vi "PQfetchResultDataNotrans.vi"(8 "error in":errorcluster, 10 "res":u64, 11 "conn":u64) -> (0 "error out":errorcluster, 1 "Data":string[][](array[string]), 2 "res_out":u64, 3 "conn_out":u64, 4 "PQnFields":i64, 6 "PQnTuples":i64)   [LabVIEW 2019, in "libpqutility64.lvlib"]
doc: "Fetch Result Data from DatabaseRequest into String Array.\nSee PostgreSQL c-lib doku for further information."
uses:
  libpqutility64.lvlib
  libpqlv64/libpqlv64.lvlib
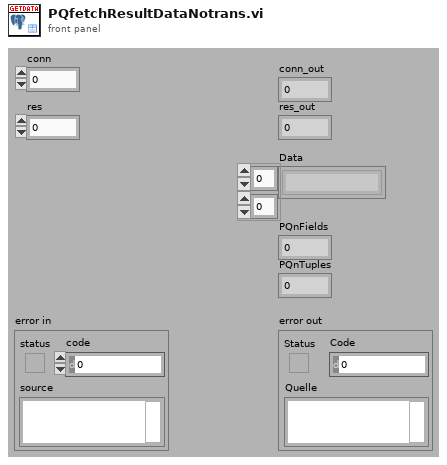
[diagram p1: front panel]
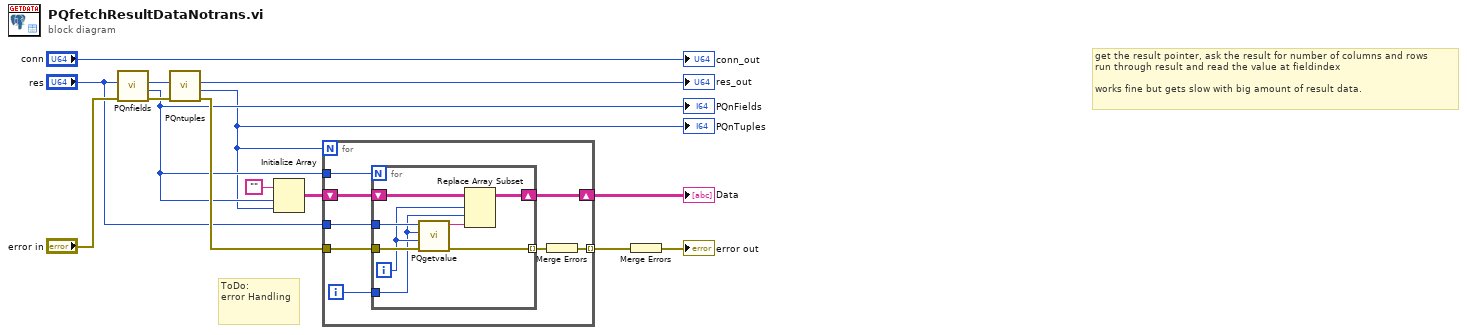
[diagram p0: block diagram]
diagram:
  # "ToDo:\nerror Handling"
  # "get the result pointer, ask the result for number of columns and rows\nrun through result and read the value at fieldindex\n\nworks fine but gets slow with big amount of result data."
  n1 = call "PQnfields.vi"("error in (no error)"="error in", "res"="res") -> ("error out"=w12:errorcluster, "PQnFields"=w6:i64, "res out"=w3:u64)  [unwired: 7 in]
  "PQnFields" <- w6
  n2 = call "PQntuples.vi"("error in (no error)"=w12, "res"=w3) -> ("error out"=w11:errorcluster, "PQnTuples"=w5:i64, "res out"=→"res_out":u64)  [unwired: 7 in]
  "PQnTuples" <- w5
  n3 = Initialize Array("", w6, w5) -> (w8:string[][])
  n4 = for {
    N: w5 -> [_]
    tunnel: "res" -> [w22]
    tunnel: w6 -> [w19]
    tunnel: w11 -> [w20]
    tunnel: [w15] -> w1 mode=indexing
    shift-right: [w18] -> w7
    shift-left: w8 -> [w17]
    i -> [w21]
    n5 = for {
      N: w19 -> [_]
      tunnel: w22 -> [w30]
      tunnel: w21 -> [w26]
      tunnel: w20 -> [w29]
      tunnel: [w28] -> w16 mode=indexing
      shift-right: [w24] -> w18
      shift-left: w17 -> [w23]
      i -> [w27]
      n6 = call "PQgetvalue.vi"("error in (no error)"=w29, "column_number"=w27, "row_number"=w26, "res"=w30) -> ("error out"=w28:errorcluster, "field_value"=w25:string)  [unwired: 6 in]
      n7 = Replace Array Subset(array=w23, new element=w25, index (row)=w27, index (col)=w26) -> (w24:string[][])
    }
    n8 = Merge Errors(w16) -> (w15:errorcluster)
  }
  "Data" <- w7
  n9 = Merge Errors(w1) -> (→"error out":errorcluster)
  "conn_out" <- "conn"
